vi "MCSC_4CH_4.03.vi"() -> ()   [LabVIEW 2012]
uses:
  <vilib>/Analysis/baseanly.llb/Mean (DBL).vi
  Libraries and VIs/Scalar_Data_4.vi
  Libraries and VIs/Scalar_Data_3.vi
  Libraries and VIs/Scalar_Data_2.vi
  Libraries and VIs/Scalar_Data.vi
  AmcsUsb.dll
  <vilib>/Analysis/NI_AALBase.lvlib
panel:
  in  "Data Reads":i32=20
  out "Loop Count":i32=19
  in  "TC Start":i32=100 min=100 max=1894
  in  "TC Length":i32=1894 min=100 max=1894
  out "Total Counts":cluster{dbl, dbl, dbl, dbl}(graph)={310512.0, 13319.0, 68145.0, 62373.0}
  out "return type":i32
  out "Raw Uncorrected Return":dbl[][](graph)
  in  "stop":bool
  out "Corrected Return":dbl[][](graph) caption="Corrected Signal"
  out "Max. Rep. Rate (Hz)":dbl=9924.573243350536
  out "Data Collection Time per Column":dbl=0.9976
  out "Minimum Sync Pulse Period(µs)":dbl=100.76 format="%.2f"
  in  "y units":u16(ring) items=["Bin #", "Sampling Time(µs)", "Range(m)"]
  in  "Time Resolution Per Bin(ns)":u16=50 min=5 max=1063 step=1
  in  "Number of Accumulates":u32=10000 min=1 max=32767 step=1
  in  "Number of Bins":u32=1995 min=2 max=4095 step=1
  in  "Pulse A Polarity":enum16{"Low", "High"}(ring)=enum."High"
  in  "Sync Pulse Polarity":enum32{"Low", "High"}(ring)=enum."High"
  in  "Accumulation Delay(ns)":u16=10 min=10 max=1270 step=1
  in  "Pulse B Delay(ns)":u32=170000 min=80 max=327600 step=1
  in  "Pulse A Delay(ns)":u32=1040 min=80 max=327600
  in  "bins":u32=1995 min=2 max=4095 step=1
  out "y offset":u16=10
  in  "ns scale":u16=50
  in  "Pulse B Polarity":enum16{"Low", "High"}(ring)=enum."High"
  out "Running?":bool
  out "Device ID":u32
  out "Open?":bool=TRUE
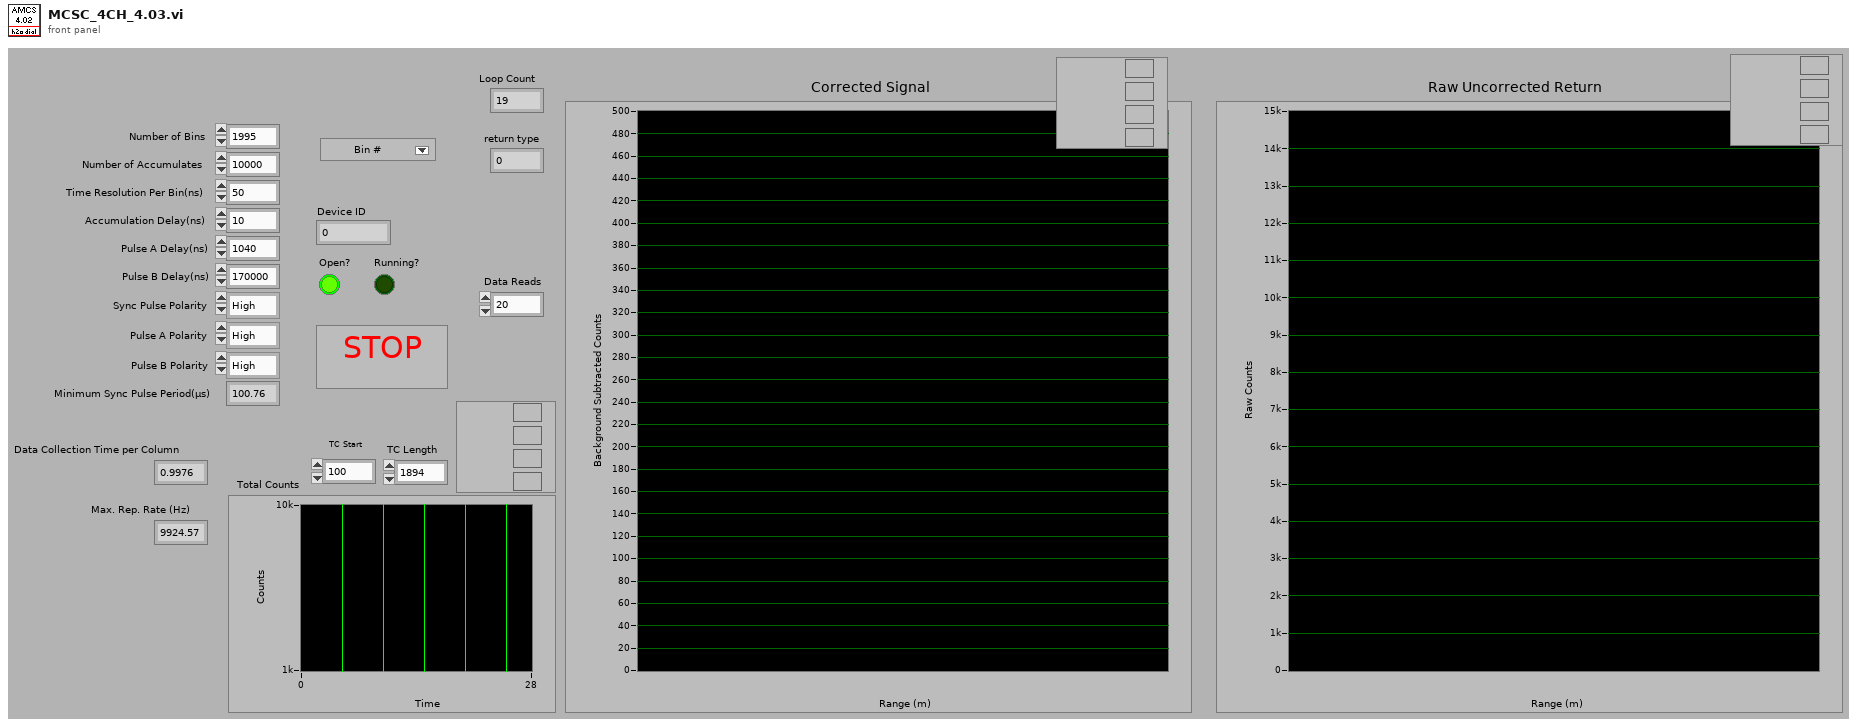
[diagram p1: front panel]
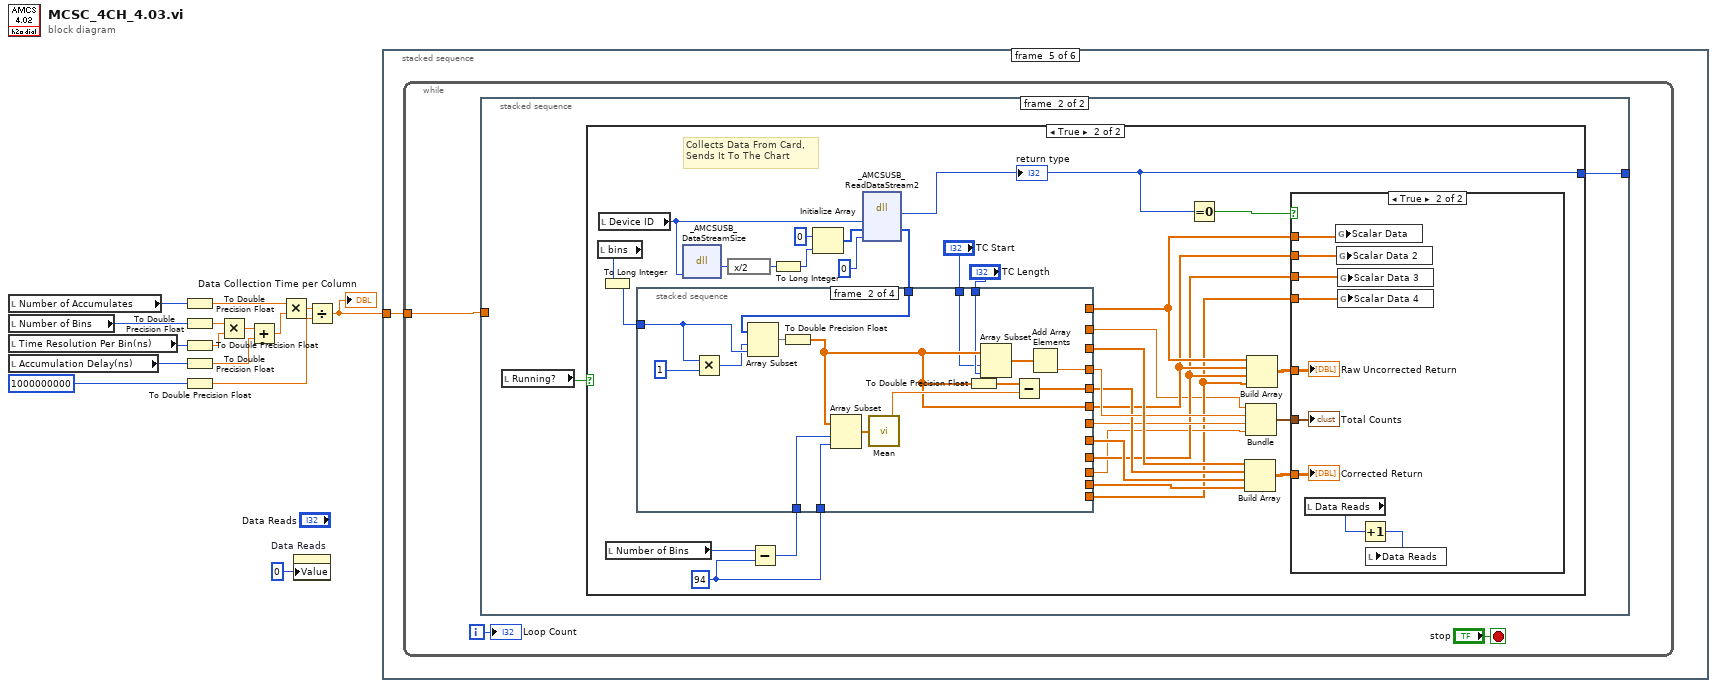
[diagram p0: block diagram]
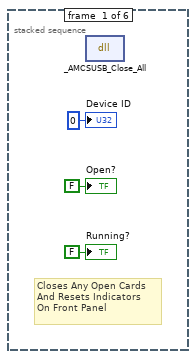
[diagram p2: hidden frame]
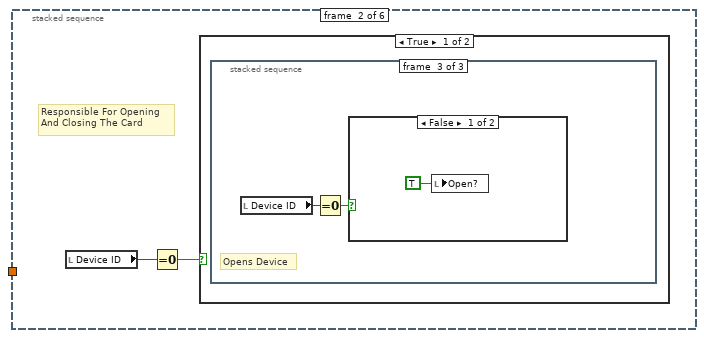
[diagram p3: hidden frame]
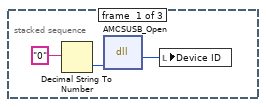
[diagram p4: hidden frame]
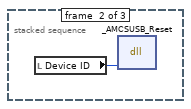
[diagram p5: hidden frame]
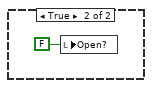
[diagram p6: hidden frame]
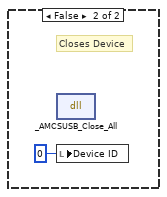
[diagram p7: hidden frame]
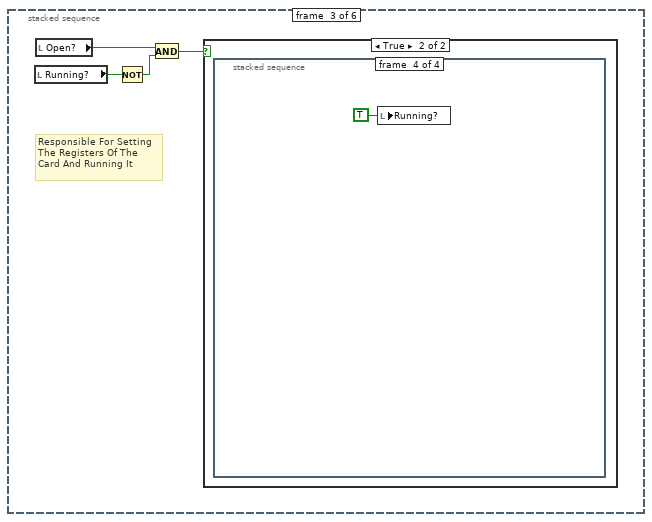
[diagram p8: hidden frame]
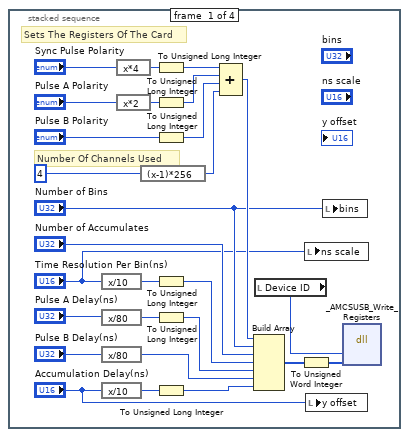
[diagram p10: hidden frame]
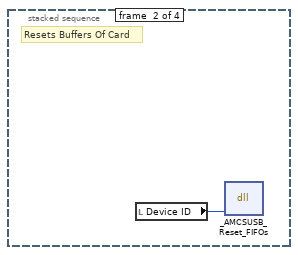
[diagram p11: hidden frame]
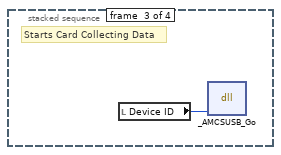
[diagram p12: hidden frame]
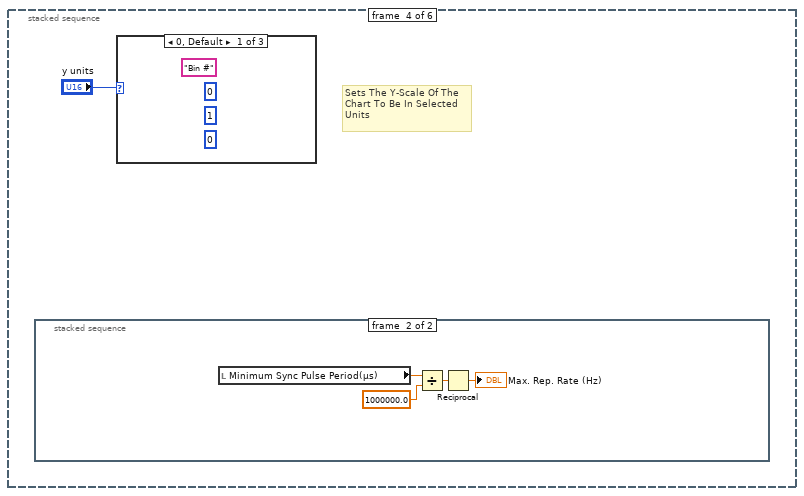
[diagram p13: hidden frame]
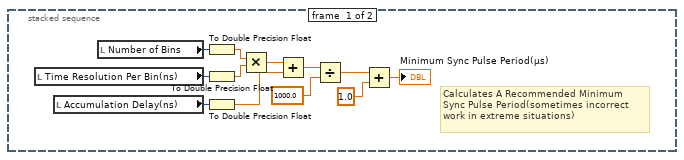
[diagram p14: hidden frame]
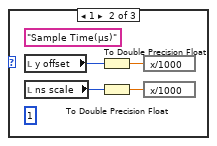
[diagram p15: hidden frame]
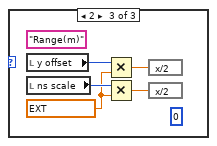
[diagram p16: hidden frame]
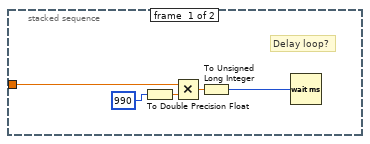
[diagram p17: hidden frame]
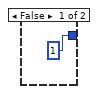
[diagram p18: hidden frame]
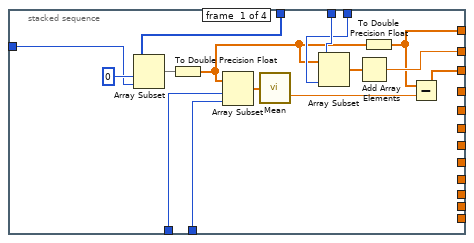
[diagram p20: hidden frame]
diagram:
  n1 = local read "Number of Accumulates"() -> (w11:u32)
  n2 = local read "Number of Bins"() -> (w6:u32)
  n3 = local read "Time Resolution Per Bin(ns)"() -> (w4:u16)
  n4 = local read "Accumulation Delay(ns)"() -> (w2:u16)
  n5 = To Double Precision Float(number=w11) -> (double precision float=w10:dbl)
  n6 = To Double Precision Float(number=w6) -> (double precision float=w5:dbl)
  n7 = To Double Precision Float(number=w4) -> (double precision float=w7:dbl)
  n8 = To Double Precision Float(number=w2) -> (double precision float=w3:dbl)
  n9 = To Double Precision Float(number=1000000000) -> (double precision float=w8:dbl)
  n10 = Multiply(x=w5, y=w7) -> (x*y=w15:dbl)
  n11 = Add(x=w15, y=w3) -> (x+y=w14:dbl)
  n12 = Multiply(x=w10, y=w14) -> (x*y=w13:dbl)
  n13 = property on="Data Reads" class="DigNum (strict)"("Value"=0 ("Data Reads")) -> ()  [unwired: 2 in, 2 out]
  n14 = Divide(x=w13, y=w8) -> (x/y=w12:dbl)
  "Data Collection Time per Column" <- w12
  n15 = stacked-sequence {
    tunnel: w12 -> [_ _ _ _ w90 _]
    frame #0 {
      # "Closes Any Open Cards\nAnd Resets Indicators\nOn Front Panel"
      n16 = dll-call lib="AmcsUsb.dll" fn="_AMCSUSB_Close_All" label="Close_All"() -> ()  [unwired: 4 in, 2 out]
      "Open?" <- FALSE ("Open?")
      "Device ID" <- u32 0 ("Device ID")
      "Running?" <- FALSE ("Running?")
    }
    frame #1 {
      # "Responsible For Opening\nAnd Closing The Card"
      n17 = local read "Device ID"() -> (w20:u32)
      n18 = Equal To 0?(x=w20) -> (x = 0?=w19:bool)
      n19 = case shown="True" w19 {
        frame True {
          # "Opens Device"
          n20 = stacked-sequence {
            frame #0 {
              n21 = Decimal String To Number(string="0" ("Device Number")) -> (number=w21:i32)  [unwired: 2 in, 1 out]
              n22 = dll-call lib="AmcsUsb.dll" fn="AMCSUSB_Open"("devnum"=w21) -> ("return type"=w22:u32)  [unwired: 4 in, 2 out]
              n23 = local write "Device ID"(w22) -> ()
            }
            frame #1 {
              n24 = local read "Device ID"() -> (w24:u32)
              n25 = dll-call lib="AmcsUsb.dll" fn="_AMCSUSB_Reset" label="Reset"("handle"=w24) -> ()  [unwired: 5 in, 2 out]
            }
            frame #2 {
              n26 = local read "Device ID"() -> (w25:u32)
              n27 = Equal To 0?(x=w25) -> (x = 0?=w26:bool)
              n28 = case shown="False" w26 {
                frame False {
                  n29 = local write "Open?"(TRUE ("Open?")) -> ()
                }
                frame True {
                  n30 = local write "Open?"(FALSE ("Open?")) -> ()
                }
              }
            }
          }
        }
        frame False {
          # "Closes Device"
          n31 = dll-call lib="AmcsUsb.dll" fn="_AMCSUSB_Close_All" label="Close_All"() -> ()  [unwired: 4 in, 2 out]
          n32 = local write "Device ID"(u32 0 ("Device ID")) -> ()
        }
      }
    }
    frame #2 {
      # "Responsible For Setting\nThe Registers Of The\nCard And Running It"
      n33 = local read "Running?"() -> (w32:bool)
      n34 = local read "Open?"() -> (w33:bool)
      n35 = Not(x=w32) -> (.not. x?=w31:bool)
      n36 = And(x=w33, y=w31) -> (x .and. y?=w30:bool)
      n37 = case shown="True" w30 {
        frame False {
        }
        frame True {
          n38 = stacked-sequence {
            frame #0 {
              # "Sets The Registers Of The Card"
              # "Number Of Channels Used"
              n39 = expression code="x/10"("Time Resolution Per Bin(ns)") -> (w37:u16)
              n40 = expression code="x/80"("Pulse A Delay(ns)") -> (w39:u32)
              n41 = expression code="x/80"("Pulse B Delay(ns)") -> (w60:u32)
              n42 = expression code="x/10"("Accumulation Delay(ns)") -> (w41:u16)
              n43 = expression code="x*4"("Sync Pulse Polarity") -> (w46:enum32{"Low", "High"})
              n44 = expression code="x*2"("Pulse A Polarity") -> (w45:enum16{"Low", "High"})
              n45 = expression code="(x-1)*256"(u32 4 ("Number of Channels Used")) -> (w54:u32)
              n46 = To Unsigned Long Integer(number=w46) -> (unsigned 32bit integer=w47:u32)
              n47 = To Unsigned Long Integer(number=w45) -> (unsigned 32bit integer=w44:u32)
              n48 = To Unsigned Long Integer(number="Pulse B Polarity") -> (unsigned 32bit integer=w42:u32)
              n49 = To Unsigned Long Integer(number=w37) -> (unsigned 32bit integer=w36:u32)
              n50 = To Unsigned Long Integer(number=w39) -> (unsigned 32bit integer=w38:u32)
              n51 = To Unsigned Long Integer(number=w41) -> (unsigned 32bit integer=w40:u32)
              n52 = Compound Arithmetic op=ADD(w47, w44, w42, w54) -> (w59:u32)
              n53 = Build Array(w59, "Number of Bins", "Number of Accumulates", w36, w38, w60, w40) -> (w35:u32[])
              n54 = local read "Device ID"() -> (w52:u32)
              n55 = To Unsigned Word Integer(number=w35) -> (unsigned 16bit integer=w34:u16[])
              n56 = local write "ns scale"("Time Resolution Per Bin(ns)") -> ()
              n57 = local write "y offset"("Accumulation Delay(ns)") -> ()
              n58 = local write "bins"("Number of Bins") -> ()
              n59 = dll-call lib="AmcsUsb.dll" fn="_AMCSUSB_Write_Registers" label="Write_Registers"("handle"=w52, "registers"=w34) -> ()  [unwired: 6 in, 2 out]
            }
            frame #1 {
              # "Resets Buffers Of Card"
              n60 = local read "Device ID"() -> (w61:u32)
              n61 = dll-call lib="AmcsUsb.dll" fn="_AMCSUSB_Reset_FIFOs" label="Reset_FIFOs"("handle"=w61) -> ()  [unwired: 5 in, 2 out]
            }
            frame #2 {
              # "Starts Card Collecting Data"
              n62 = local read "Device ID"() -> (w62:u32)
              n63 = dll-call lib="AmcsUsb.dll" fn="_AMCSUSB_Go" label="Go"("handle"=w62) -> ()  [unwired: 5 in, 2 out]
            }
            frame #3 {
              n64 = local write "Running?"(TRUE) -> ()
            }
          }
        }
      }
    }
    frame #3 {
      # "Sets The Y-Scale Of The\nChart To Be In Selected\nUnits"
      n65 = stacked-sequence {
        frame #0 {
          # "Calculates A Recommended Minimum\nSync Pulse Period(sometimes incorrect\nwork in extreme situations)"
          n66 = local read "Time Resolution Per Bin(ns)"() -> (w71:u16)
          n67 = local read "Accumulation Delay(ns)"() -> (w73:u16)
          n68 = local read "Number of Bins"() -> (w72:u32)
          n69 = To Double Precision Float(number=w72) -> (double precision float=w74:dbl)
          n70 = To Double Precision Float(number=w71) -> (double precision float=w75:dbl)
          n71 = To Double Precision Float(number=w73) -> (double precision float=w76:dbl)
          n72 = Multiply(x=w74, y=w75) -> (x*y=w70:dbl)
          n73 = Add(x=w70, y=w76) -> (x+y=w68:dbl)
          n74 = Divide(x=w68, y=1000.0) -> (x/y=w67:dbl)
          n75 = Add(x=w67, y=1.0) -> (x+y=→"Minimum Sync Pulse Period(µs)":dbl)
        }
        frame #1 {
          n76 = local read "Minimum Sync Pulse Period(µs)"() -> (w78:dbl)
          n77 = Divide(x=w78, y=1000000.0) -> (x/y=w77:dbl)
          n78 = Reciprocal(x=w77) -> (1/x=→"Max. Rep. Rate (Hz)":dbl)
        }
      }
      n79 = case shown="0, Default" "y units" {
        frame 0, Default {
          (unwired) u8 0 ("Y Scale.Format & Precision:Precision")
          (unwired) u16 1 ("Y Scale.Offset and Multiplier:Multiplier")
          (unwired) "Bin #" ("Y Scale.Name Label.Text")
          (unwired) u16 0 ("Y Scale.Offset and Multiplier:Offset")
        }
        frame 1 {
          (unwired) u8 1 ("Y Scale.Format & Precision:Precision")
          (unwired) "Sample Time(µs)" ("Y Scale.Name Label.Text")
          n80 = local read "y offset"() -> (w84:u16)
          n81 = local read "ns scale"() -> (w83:u16)
          n82 = To Double Precision Float(number=w84) -> (double precision float=w82:dbl)
          n83 = To Double Precision Float(number=w83) -> (double precision float=w81:dbl)
          n84 = expression code="x/1000"(w82) -> ()  [unwired: 1 out]
          n85 = expression code="x/1000"(w81) -> ()  [unwired: 1 out]
        }
        frame 2 {
          (unwired) u8 0 ("Y Scale.Format & Precision:Precision")
          w85 = ext 0.299792458 ("y")
          (unwired) "Range(m)" ("Y Scale.Name Label.Text")
          n86 = local read "y offset"() -> (w88:u16)
          n87 = local read "ns scale"() -> (w89:u16)
          n88 = Multiply(x=w88, y=w85) -> (x*y=w87:ext)
          n89 = Multiply(x=w89, y=w85) -> (x*y=w86:ext)
          n90 = expression code="x/2"(w87) -> ()  [unwired: 1 out]
          n91 = expression code="x/2"(w86) -> ()  [unwired: 1 out]
        }
      }
    }
    frame #4 {
      n92 = while {
        tunnel: w90 -> [w93]
        i -> [w91]
        stop <- "stop" stop-if-true
        n93 = stacked-sequence {
          tunnel: w93 -> [w98 _]
          tunnel: [_ w99] -> _
          frame #0 {
            # "Delay loop?"
            n94 = To Double Precision Float(number=990) -> (double precision float=w96:dbl)
            n95 = Multiply(x=w98, y=w96) -> (x*y=w95:dbl)
            n96 = To Unsigned Long Integer(number=w95) -> (unsigned 32bit integer=w94:u32)
            n97 = Wait (ms)(milliseconds to wait=w94) -> ()  [unwired: 1 out]
          }
          frame #1 {
            n98 = local read "Running?"() -> (w100:bool)
            n99 = case shown="True" w100 {
              tunnel: [1 ("return type") w102] -> w99
              frame False {
              }
              frame True {
                w117 = 94 ("length")
                # "Collects Data From Card,\nSends It To The Chart"
                n100 = local read "bins"() -> (w122:u32)
                n101 = local read "Device ID"() -> (w130:u32)
                n102 = To Long Integer(number=w122) -> (32bit integer=w121:i32)
                n103 = local read "Number of Bins"() -> (w119:u32)
                n104 = dll-call lib="AmcsUsb.dll" fn="_AMCSUSB_DataStreamSize" label="DataStreamSize"("handle"=w130) -> ("return type"=w129:u16)  [unwired: 4 in, 2 out]
                n105 = expression code="x/2"(w129) -> (w128:u16)
                n106 = Subtract(x=w119, y=w117) -> (x-y=w118:u32)
                n107 = To Long Integer(number=w128) -> (32bit integer=w127:i32)
                n108 = Initialize Array(u32 0 ("element"), w127) -> (w131:u32[])
                n109 = dll-call lib="AmcsUsb.dll" fn="_AMCSUSB_ReadDataStream2" label="ReadDataStream2"("handle"=w130, "buffer"=w131, "BytesReturned"=u32 0) -> ("return type"=w102:i32, "buffer"=w123:u16[])  [unwired: 5 in, 2 out]
                "return type" <- w102
                n110 = stacked-sequence {
                  tunnel: w123 -> [w156 w173 w189 w205]
                  tunnel: w121 -> [w155 w161 w181 w197]
                  tunnel: [w144 _ _ _] -> w120
                  tunnel: [w143 _ _ _] -> w114
                  tunnel: w118 -> [w152 w169 w185 w201]
                  tunnel: w117 -> [w151 w170 w186 w202]
                  tunnel: [w149 _ _ _] -> w104
                  tunnel: "TC Start" -> [w148 w158 w174 w190]
                  tunnel: "TC Length" -> [w147 w159 w175 w191]
                  tunnel: [_ w167 _ _] -> w113
                  tunnel: [_ w164 _ _] -> w112
                  tunnel: [_ w163 _ _] -> w111
                  tunnel: [_ _ w178 _] -> w110
                  tunnel: [_ _ w177 _] -> w109
                  tunnel: [_ _ w176 _] -> w108
                  tunnel: [_ _ _ w194] -> w106
                  tunnel: [_ _ _ w193] -> w107
                  tunnel: [_ _ _ w192] -> w105
                  frame #0 {
                    n111 = Array Subset(array=w156, index=0 ("dimension size"), length=w155) -> (w153:u16[])
                    n112 = To Double Precision Float(number=w153) -> (double precision float=w146:dbl[])
                    n113 = Array Subset(array=w146, index=w152, length=w151) -> (w154:dbl[])
                    n114 = call-poly <vilib>:"Mean.vi"("X"=w154) -> ("mean"=w145:dbl)  [unwired: 1 out]
                    n115 = Array Subset(array=w146, index=w148, length=w147) -> (w150:dbl[])
                    n116 = Add Array Elements(numeric array=w150) -> (sum=w149:dbl)
                    n117 = To Double Precision Float(number=w146) -> (double precision float=w144:dbl[])
                    n118 = Subtract(x=w144, y=w145) -> (x-y=w143:dbl[])
                  }
                  frame #1 {
                    n119 = Multiply(x=w161, y=1 ("Far Input Ch")) -> (x*y=w160:i32)
                    n120 = Array Subset(array=w173, index=w160, length=w161) -> (w172:u16[])
                    n121 = To Double Precision Float(number=w172) -> (double precision float=w163:dbl[])
                    n122 = Array Subset(array=w163, index=w169, length=w170) -> (w171:dbl[])
                    n123 = call-poly <vilib>:"Mean.vi"("X"=w171) -> ("mean"=w165:dbl)  [unwired: 1 out]
                    n124 = To Double Precision Float(number=w163) -> (double precision float=w166:dbl[])
                    n125 = Array Subset(array=w163, index=w158, length=w159) -> (w168:dbl[])
                    n126 = Subtract(x=w166, y=w165) -> (x-y=w164:dbl[])
                    n127 = Add Array Elements(numeric array=w168) -> (sum=w167:dbl)
                  }
                  frame #2 {
                    n128 = Multiply(x=w181, y=2 ("Far Input Ch")) -> (x*y=w180:i32)
                    n129 = Array Subset(array=w189, index=w180, length=w181) -> (w188:u16[])
                    n130 = To Double Precision Float(number=w188) -> (double precision float=w176:dbl[])
                    n131 = Array Subset(array=w176, index=w185, length=w186) -> (w187:dbl[])
                    n132 = call-poly <vilib>:"Mean.vi"("X"=w187) -> ("mean"=w182:dbl)  [unwired: 1 out]
                    n133 = To Double Precision Float(number=w176) -> (double precision float=w183:dbl[])
                    n134 = Array Subset(array=w176, index=w174, length=w175) -> (w184:dbl[])
                    n135 = Subtract(x=w183, y=w182) -> (x-y=w177:dbl[])
                    n136 = Add Array Elements(numeric array=w184) -> (sum=w178:dbl)
                  }
                  frame #3 {
                    n137 = Multiply(x=w197, y=3 ("Far Input Ch")) -> (x*y=w196:i32)
                    n138 = Array Subset(array=w205, index=w196, length=w197) -> (w204:u16[])
                    n139 = To Double Precision Float(number=w204) -> (double precision float=w192:dbl[])
                    n140 = Array Subset(array=w192, index=w201, length=w202) -> (w203:dbl[])
                    n141 = call-poly <vilib>:"Mean.vi"("X"=w203) -> ("mean"=w198:dbl)  [unwired: 1 out]
                    n142 = To Double Precision Float(number=w192) -> (double precision float=w199:dbl[])
                    n143 = Array Subset(array=w192, index=w190, length=w191) -> (w200:dbl[])
                    n144 = Subtract(x=w199, y=w198) -> (x-y=w193:dbl[])
                    n145 = Add Array Elements(numeric array=w200) -> (sum=w194:dbl)
                  }
                }
                n146 = Equal To 0?(x=w102) -> (x = 0?=w103:bool)
                n147 = Build Array(w114, w112, w109, w107) -> (w126:dbl[][])
                n148 = Bundle(w104, w113, w110, w106) -> (w124:cluster{dbl, dbl, dbl, dbl})  [unwired: 1 in]
                n149 = Build Array(w120, w111, w108, w105) -> (w125:dbl[][])
                n150 = case shown="True" w103 {
                  tunnel: w126 -> [_ w142]
                  tunnel: w125 -> [_ w141]
                  tunnel: w124 -> [_ w140]
                  tunnel: w120 -> [_ w137]
                  tunnel: w111 -> [_ w134]
                  tunnel: w108 -> [_ w135]
                  tunnel: w105 -> [_ w136]
                  frame False {
                  }
                  frame True {
                    n151 = local read "Data Reads"() -> (w138:i32)
                    n152 = global write "Scalar_Data.vi" "Scalar Data"(w137) -> ()
                    n153 = global write "Scalar_Data_2.vi" "Scalar Data 2"(w134) -> ()
                    n154 = global write "Scalar_Data_3.vi" "Scalar Data 3"(w135) -> ()
                    n155 = global write "Scalar_Data_4.vi" "Scalar Data 4"(w136) -> ()
                    n156 = Increment(x=w138) -> (x+1=w139:i32)
                    n157 = local write "Data Reads"(w139) -> ()
                    "Corrected Return" <- w142
                    "Raw Uncorrected Return" <- w141
                    "Total Counts" <- w140
                  }
                }
              }
            }
          }
        }
        "Loop Count" <- w91
      }
    }
    frame #5 {
      # "Closes Any Open Cards\nAnd Resets Indicators\nOn Front Panel"
      n158 = dll-call lib="AmcsUsb.dll" fn="_AMCSUSB_Close_All" label="Close_All"() -> ()  [unwired: 4 in, 2 out]
      n159 = local write "Device ID"(u32 0 ("Device ID")) -> ()
      n160 = local write "Open?"(TRUE ("Open?")) -> ()
      n161 = local write "Running?"(FALSE ("Running?")) -> ()
    }
  }
